vi "Create myTemp.vi"(8 "error in (no error)":errorcluster, 10 "device name (myDAQ1)":tag="myDAQ1") -> (0 "error out":errorcluster, 3 "task array out":refnum<k21>[](array[refnum]))   [LabVIEW 2013]
doc: "This VI creates the DAQmx tasks needed to run the PITSCO myTemp.\n\nThe PITSCO myTemp miniSystem uses 2 DAQmx Tasks.\nTask0: Analog Input 0:1\nTask1: Digital Output 0:2, 5:7\n\nDigital Outputs 0,1,2 control the MUX for AI0\nDigital Outputs 5,6,7 control the MUX for AI1\n\n If the Aux switch on the device is in the MUX position you can read all 7 temperatures. If the switch is in the AUX position then AI1 will read directly from the myTemp AI1 screw terminal."
uses:
  <vilib>/DAQmx/create/channels.llb/DAQmx Create Channel (DO-Digital Output).vi
  <vilib>/DAQmx/create/channels.llb/DAQmx Create Channel (AI-Voltage-Basic).vi
  <vilib>/DAQmx/configure/timing.llb/DAQmx Timing (Sample Clock).vi
  <resource>/objmgr/daqmx.rc
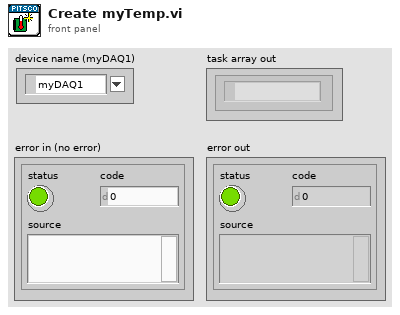
[diagram p1: front panel]
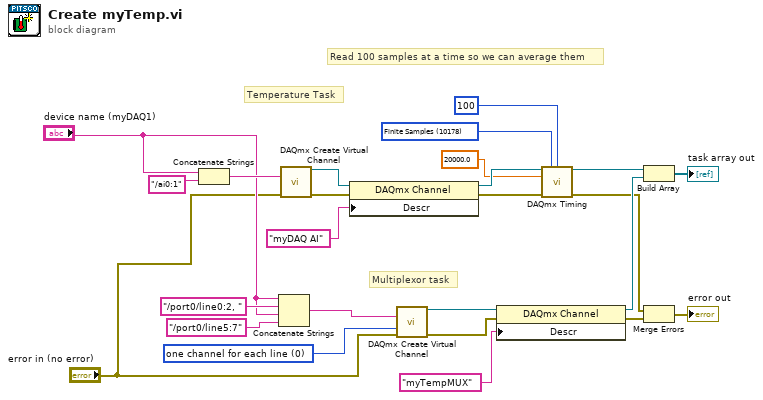
[diagram p0: block diagram]
diagram:
  w21 = 0 items=["one channel for each line", "one channel for all lines"] ("line grouping (1 chan for each line)")
  w9 = 10178 items=["Finite Samples"=10178, "Continuous Samples"=10123, "Hardware Timed Single Point"=12522] ("sample mode (Finite.)")
  # "Read 100 samples at a time so we can average them"
  # "Temperature Task"
  # "Multiplexor task"
  n1 = Concatenate Strings("device name (myDAQ1)", "/ai0:1" ("string")) -> (w16:string)
  n2 = Concatenate Strings("device name (myDAQ1)", "/port0/line0:2, " ("string"), "device name (myDAQ1)", "/port0/line5:7" ("string")) -> (w23:string)
  n3 = call-poly <vilib>:"DAQmx Create Virtual Channel.vi"("physical channels"=w16, "error in"="error in (no error)") -> ("task out"=w11:refnum<k21>, "error out"=w13:errorcluster)  [unwired: 12 in]
  n4 = property class="DAQmx Channel"(reference=w11, error in=w13, "Descr"="myDAQ AI" ("Descr (myDAQ AI)")) -> (reference out=w12:refnum<k21>, error out=w14:errorcluster)
  n5 = call-poly <vilib>:"DAQmx Create Virtual Channel.vi"("lines"=w23, "line grouping"=w21, "error in"="error in (no error)") -> ("task out"=w19:refnum<k21>, "error out"=w20:errorcluster)  [unwired: 11 in]
  n6 = property class="DAQmx Channel"(reference=w19, error in=w20, "Descr"="myTempMUX" ("Channel Description")) -> (reference out=w24:refnum<k21>, error out=w25:errorcluster)
  n7 = call-poly <vilib>:"DAQmx Timing.vi"("task/channels in"=w12, "sample mode"=w9, "samples per channel"=100 ("samples per channel(100)"), "rate"=20000.0 ("rate (1kHz)"), "error in"=w14) -> ("task out"=w17:refnum<k21>, "error out"=w18:errorcluster)  [unwired: 9 in]
  n8 = Build Array(w17, w24) -> (→"task array out":refnum<k21>[])
  n9 = Merge Errors(w18, w25) -> (→"error out":errorcluster)
